vi "Data to CSV Line.vi"(8 "error in (no error)":errorcluster, 10 "Elapsed Time":string, 11 "Array":waveform(dbl)[](array[waveform])) -> (0 "error out":errorcluster, 2 "Spreadsheet String":string[](array[string]))   [LabVIEW 2018, in "CSV Log.lvlib"]
uses:
  CSV Log.lvlib
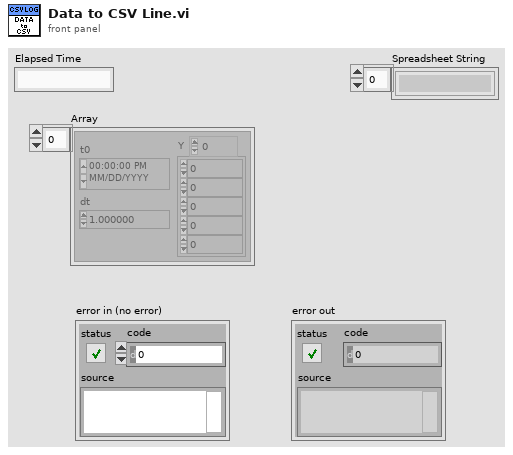
[diagram p1: front panel]
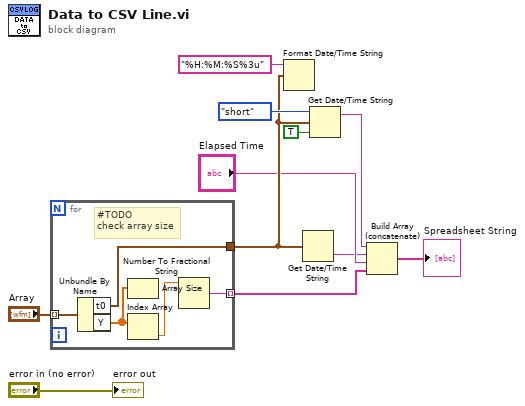
[diagram p0: block diagram]
diagram:
  n1 = for {
    tunnel: "Array" -> [w16] mode=indexing
    tunnel: [w13] -> w5 mode=indexing
    tunnel: [w12] -> w4
    # "#TODO\ncheck array size"
    n2 = Unbundle By Name(w16) -> ("t0"=w12:timestamp, "Y"=w15:dbl[])
    n3 = Array Size(array=w15) -> ()  [unwired: 1 out]
    n4 = Index Array(array=w15) -> (element=w14:dbl)  [unwired: 1 in]
    n5 = Number To Fractional String(number=w14) -> (F-format string=w13:string)  [unwired: 3 in]
  }
  n6 = Format Date/Time String(time format string (%c)="%H:%M:%S%3u", seconds (now)=w4) -> ()  [unwired: 1 in, 1 out]
  n7 = Get Date/Time String(seconds (now)=w4) -> (time string=w1:string)  [unwired: 2 in, 1 out]
  n8 = Get Date/Time String(date format (0)=enum16{"short", "long", "abbreviated"}."short", seconds (now)=w4, want seconds? (F)=TRUE) -> (date string=w6:string)  [unwired: 1 out]
  n9 = Build Array (concatenate)(w6, w1, "Elapsed Time", w5) -> (→"Spreadsheet String":string[])
  "error out" <- "error in (no error)"
